vi "WPI_DashboardLogging Global.vi"() -> ()   [LabVIEW 2017]
uses:
  <vilib>/Rock Robotics/WPI/Dashboard/WPI_DashboardPlay Operation.ctl
  <vilib>/Rock Robotics/Network Tables/NT Event Type.ctl
  <vilib>/Rock Robotics/Network Tables/Protocol Operations.ctl
  <vilib>/Rock Robotics/Network Tables/Field Data.ctl
  <vilib>/Rock Robotics/Network Tables/Field Type.ctl
  <vilib>/Rock Robotics/Network Tables/Sequence.ctl
panel:
  in  "Display Names":string[](array[string])
  in  "Video Frame #":T1
  in  "Binding Event Ref":refnum<user-event>
  in  "Codec Name":string="Motion JPEG (NI Vision)"
  in  "Scrollbar":refnum<vi>
  in  "Speed":T2(ring)
  in  "Operation":T3
  in  "Logging Filename":path=path "testLog.ntl"
  in  "Recording":enum32{"Stop", "Record", "Playback"}(radio)
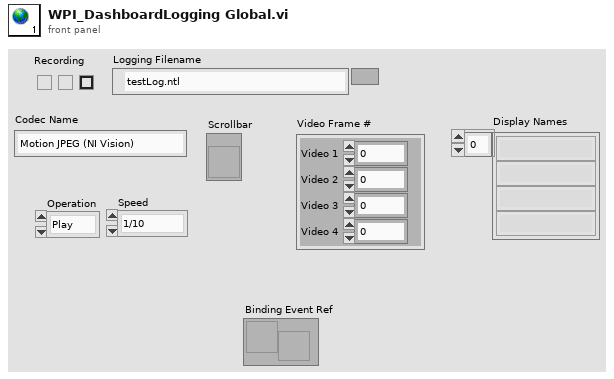
[diagram p1: front panel]
types:
  T1 = cluster{"Video 1":i32, "Video 2":i32, "Video 3":i32, "Video 4":i32}
  T2 = enum16{"1/10", "1/5", "1/2", "1", "2", "5", "10"}
  T3 = typedef "WPI_DashboardPlay Operation.ctl" = enum16{"Play", "Pause", "Finished"}
diagram:
